vi "GetDefaultValues.vi"() -> (2 "Default Values":string[](array[string]))   [LabVIEW 2019, in "ResultTree.lvclass"]
uses:
  ResultTree.lvclass
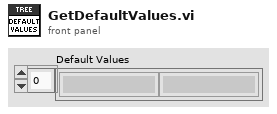
[diagram p1: front panel]
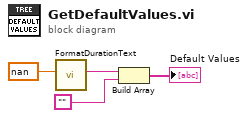
[diagram p0: block diagram]
diagram:
  n1 = call "FormatDurationText.vi"("Duration [s]"=nan) -> ("String"=w3:string)  [unwired: 10 in]
  n2 = Build Array(w3, "") -> (→"Default Values":string[])
